vi "write_attributes.vi"(8 "error in (no error)":errorcluster, 10 "attributes":T1, 11 "BayesianRidge in":refnum<class "BayesianRidge.lvclass">) -> (0 "error out":errorcluster, 3 "BayesianRidge out":refnum<class "BayesianRidge.lvclass">)   [LabVIEW 2020, in "BayesianRidge.lvclass"]
uses:
  BayesianRidge.lvclass
  Controls/bayesian_ridge_attributes.ctl
  BayesianRidge.lvclass/BayesianRidge.ctl
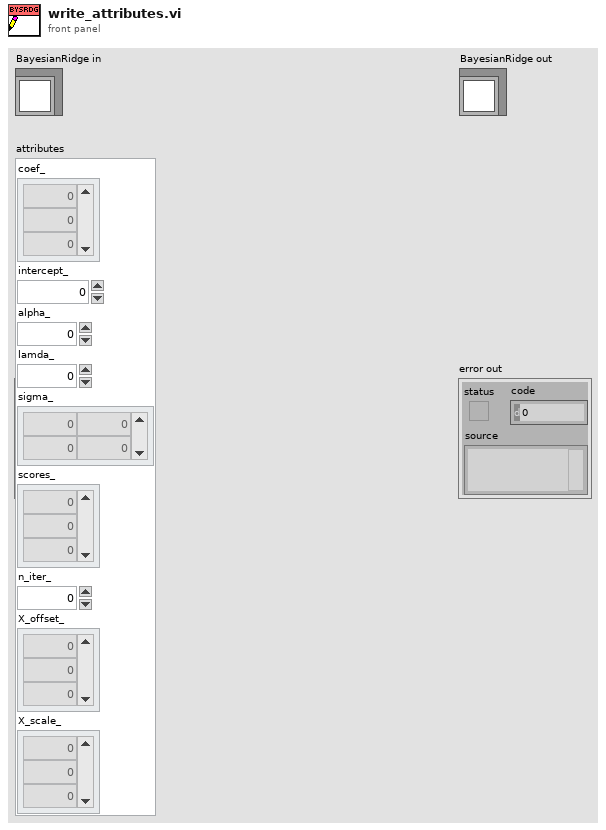
[diagram p1: front panel]
types:
  T1 = typedef "bayesian_ridge_attributes.ctl" = cluster{"coef_":dbl[], "intercept_":dbl, "alpha_":dbl, "lamda_":dbl, "sigma_":dbl[][], "scores_":dbl[], "n_iter_":dbl, "X_offset_":dbl[], "X_scale_":dbl[]}
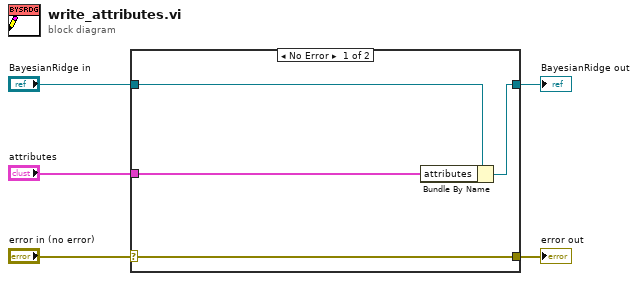
[diagram p0: block diagram]
diagram:
  n1 = case shown="No Error" "error in (no error)" {
    selector: "error in (no error)" -> [w9 w10]
    tunnel: [w9 w10] -> w4
    tunnel: [w7 w11] -> w2
    tunnel: "BayesianRidge in" -> [w8 w11]
    tunnel: "attributes" -> [w6 _]
    frame No Error {
      n2 = Bundle By Name(cluster=w8, "attributes"=w6) -> (w7:refnum<class "BayesianRidge.lvclass">)
    }
    frame Error {
    }
  }
  "error out" <- w4
  "BayesianRidge out" <- w2
